vi "SetupStrainBase.vi"(0 "Refnum in":refnum<k21>, 1 "excitation value":dbl, 2 "physical channel":string, 3 "channel name":string, 5 "minimum value":dbl, 7 "nominal gage resistance":dbl, 9 "maximum value":dbl, 11 "error in (no error)":errorcluster, 12 "custom scale name":string, 13 "gage factor":dbl, 14 "strain configuration":i32) -> (4 "Refnum out":refnum<k21>, 15 "error out":errorcluster)   [LabVIEW 2011]
uses:
  <vilib>/DAQmx/create/channels.llb/DAQmx Create Channel (AI-Strain-Strain Gage).vi
  <vilib>/DAQmx/create/channels.llb/DAQmx Create Channel (TEDS-AI-Strain-Strain Gage).vi
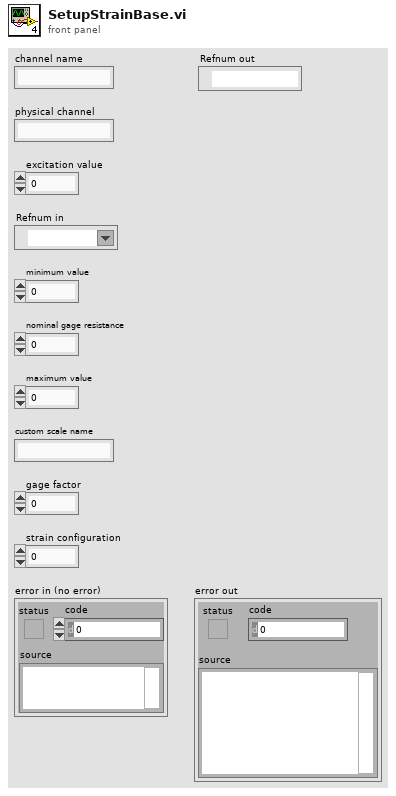
[diagram p1: front panel]
types:
  T1 = cluster{"lead resistance":dbl, "initial bridge voltage":dbl, "excitation source":i32, "excitation value":dbl}
  T2 = cluster{"gage factor":dbl, "nominal gage resistance":dbl, "poisson ratio":dbl}
  T3 = cluster{"strain configuration":i32, "lead resistance":dbl, "initial bridge voltage":dbl, "excitation source":i32, "excitation value":dbl}
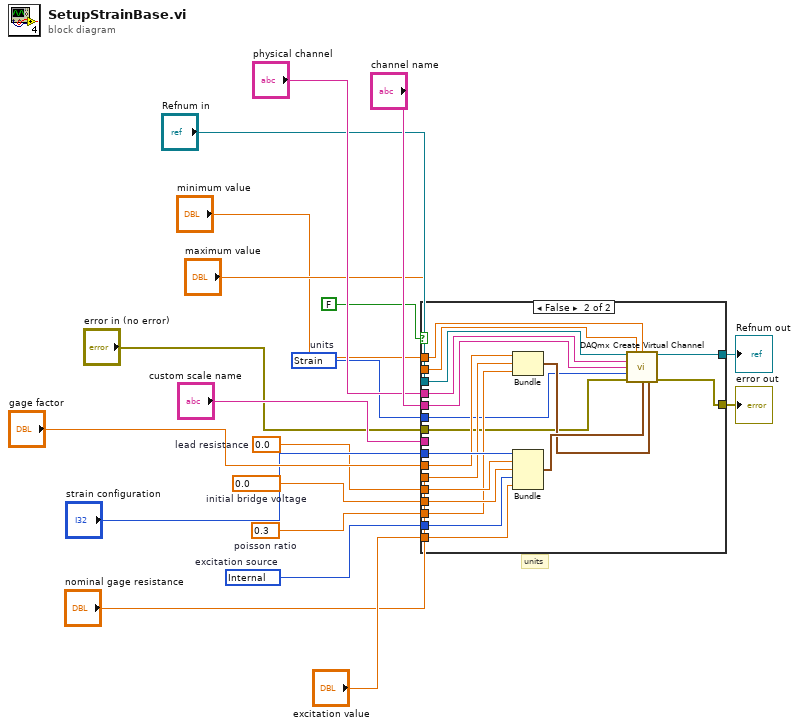
[diagram p0: block diagram]
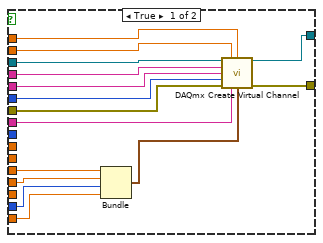
[diagram p2: hidden frame]
diagram:
  w6 = 10200 items=["Internal"=10200, "External"=10167, "None"=10230]  # excitation source
  w5 = 0.3  # poisson ratio
  w4 = 0.0  # initial bridge voltage
  w3 = 0.0  # lead resistance
  w2 = 10299 items=["Strain"=10299, "From Custom Scale"=10065]  # units
  # "units"
  n1 = case shown="False" FALSE {
    tunnel: "Refnum in" -> [w34 w53]
    tunnel: w2 -> [w26 w36]
    tunnel: [w33 w52] -> w7
    tunnel: [w32 w51] -> w8
    tunnel: "channel name" -> [w20 w39]
    tunnel: "strain configuration" -> [_ w48]
    tunnel: w3 -> [w30 w47]
    tunnel: w4 -> [w29 w46]
    tunnel: w6 -> [w28 w45]
    tunnel: "excitation value" -> [w27 w44]
    tunnel: "gage factor" -> [_ w43]
    tunnel: "nominal gage resistance" -> [_ w42]
    tunnel: w5 -> [_ w41]
    tunnel: "error in (no error)" -> [w25 w35]
    tunnel: "physical channel" -> [w21 w40]
    tunnel: "maximum value" -> [w24 w38]
    tunnel: "minimum value" -> [w23 w37]
    tunnel: "custom scale name" -> [w22 _]
    frame True {
      n2 = Bundle("lead resistance"=w30, "initial bridge voltage"=w29, "excitation source"=w28, "excitation value"=w27) -> (w31:T1)  [unwired: 1 out]
      n3 = call-poly <vilib>:"DAQmx Create Virtual Channel.vi"("task in"=w34, "maximum value"=w24, "minimum value"=w23, "physical channels"=w21, "name to assign"=w20, "units"=w26, "error in"=w25, "custom scale name"=w22, "bridge information"=w31) -> ("task out"=w33:refnum<k21>, "error out"=w32:errorcluster)  [unwired: 1 in, 4 out]
    }
    frame False {
      n4 = Bundle("gage factor"=w43, "nominal gage resistance"=w42, "poisson ratio"=w41) -> (w49:T2)  [unwired: 1 out]
      n5 = Bundle("strain configuration"=w48, "lead resistance"=w47, "initial bridge voltage"=w46, "excitation source"=w45, "excitation value"=w44) -> (w50:T3)  [unwired: 1 out]
      n6 = call-poly <vilib>:"DAQmx Create Virtual Channel.vi"("task in"=w53, "maximum value"=w38, "minimum value"=w37, "physical channels"=w40, "name to assign"=w39, "units"=w36, "error in"=w35, "bridge information"=w50, "strain gage information"=w49) -> ("task out"=w52:refnum<k21>, "error out"=w51:errorcluster)  [unwired: 1 in, 4 out]
    }
  }
  "Refnum out" <- w7
  "error out" <- w8
